vi "fgv_UI-set.vi"(7 "cmd":T1=enum."DL950 graph show", 8 "error in":errorcluster, 10 "Value":dbl, 11 "onoff":bool) -> (0 "error out":errorcluster)   [LabVIEW 2019]
uses:
  UI.ctl
  _ctrl/rw.ctl
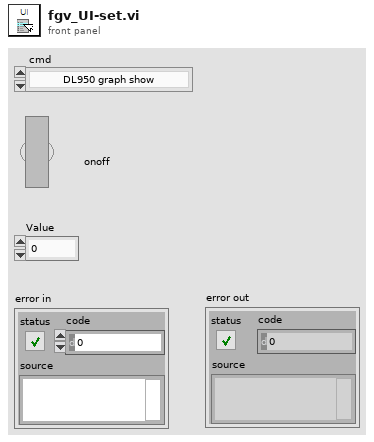
[diagram p1: front panel]
types:
  T1 = typedef "UI.ctl" = enum16{"Alarm yellow", "DL950 graph show", "DL950 graph clear", "AO value", "AO blink onoff", "Discharge relay", "Input Power", "Outpower", "Relay in1", "Relay in2", "Relay in3", "Relay in4", "Relay in5", "Relay in6", "Relay out1", "Relay out2", "Relay out3", "Relay out4", "Relay out5", "Relay out6", "Relay all off"}
  T2 = typedef "rw.ctl" = enum16{"read", "write"}
  T3 = typedef "ref_all.ctl" = cluster{"BP4610 Config":refnum<vi>, "DSP1950 Config":refnum<vi>, "2470-config":refnum<vi>, "cDAQ 9269 AO config":refnum<vi>, "cDAQ 9221 Config":refnum<vi>, "cDAQ-9467 Config":refnum<vi>, "Waveform":refnum<vi>, "DL950 wfm":refnum<vi>, "AI Graph":refnum<vi>, "AO_Wave-config":refnum<vi>, "DL950 items":refnum<vi>, "Volt":refnum<vi>, "Current":refnum<vi>, "AO_Level":refnum<vi>, "RC-Test Judgement ":refnum<vi>, "Log path":refnum<vi>, "시험명":refnum<vi>, "file renew[Hr]":refnum<vi>, "Breakdown-Spec":refnum<vi>, "paste":refnum<vi>, "copy":refnum<vi>, "DL950_config":refnum<vi>, "종료시간":refnum<vi>, "경과시간":refnum<vi>, "Apply":refnum<vi>, "DSP Config LV ":refnum<vi>, "Testconfig":refnum<vi>}
  T4 = typedef "ref.ctl" = cluster{"relay 1":refnum<vi>, "relay 2":refnum<vi>, "relay 3":refnum<vi>, "relay 4":refnum<vi>, "relay 5":refnum<vi>, "relay 6":refnum<vi>, "PoutR 1":refnum<vi>, "PoutR 2":refnum<vi>, "PoutR 3":refnum<vi>, "PoutR 4":refnum<vi>, "PoutR 5":refnum<vi>, "PoutR 6":refnum<vi>, "Discharge":refnum<vi>, "Input Pwr":refnum<vi>, "Output_HV":refnum<vi>, "AO onoff":refnum<vi>}
  T5 = typedef "ui_dev-operator.ctl" = cluster{"Operation stutus":refnum<vi>, "Test Status":refnum<vi>, "Setting":refnum<vi>, "Manual":refnum<vi>, "Main":refnum<vi>, "RCstart":refnum<vi>, "채널선택":refnum<vi>, "시험명":refnum<vi>, "Tab Control_manual":refnum<vi>, "시험 모드":refnum<vi>, "HW check":refnum<vi>, "login":refnum<vi>, "logout":refnum<vi>}
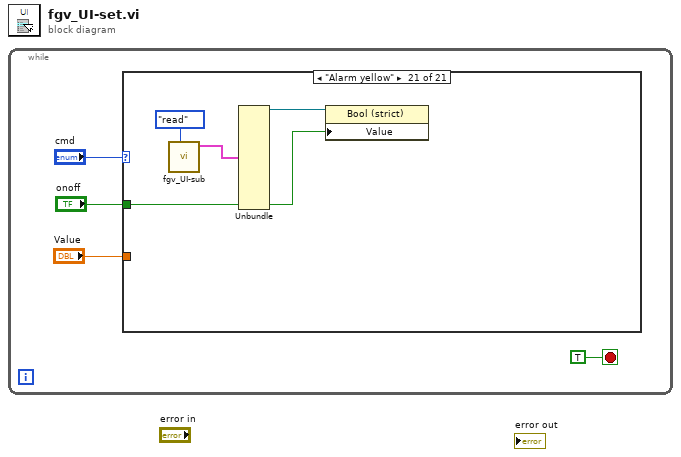
[diagram p0: block diagram]
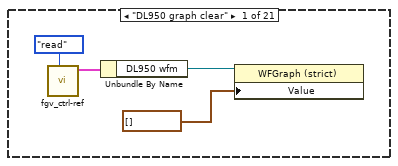
[diagram p2: hidden frame]
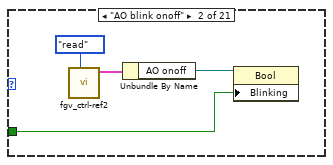
[diagram p3: hidden frame]
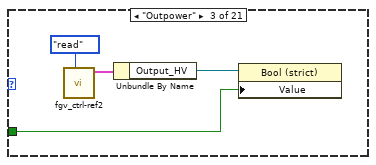
[diagram p4: hidden frame]
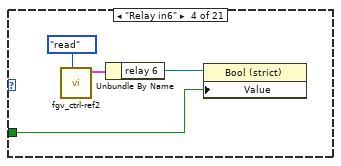
[diagram p5: hidden frame]
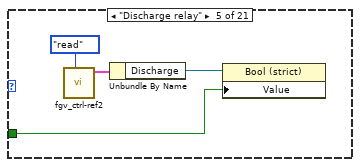
[diagram p6: hidden frame]
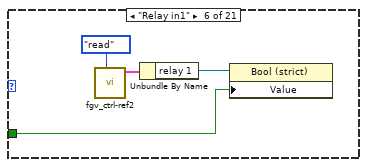
[diagram p7: hidden frame]
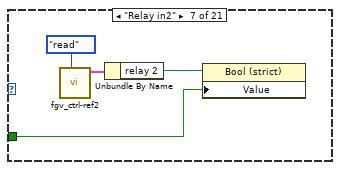
[diagram p8: hidden frame]
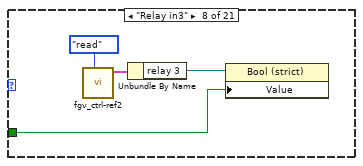
[diagram p9: hidden frame]
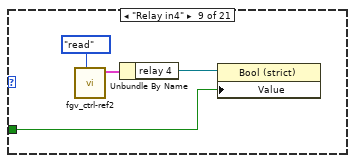
[diagram p10: hidden frame]
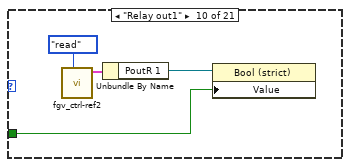
[diagram p11: hidden frame]
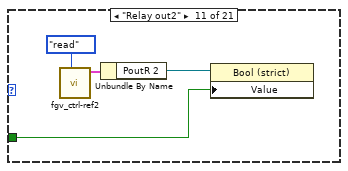
[diagram p12: hidden frame]
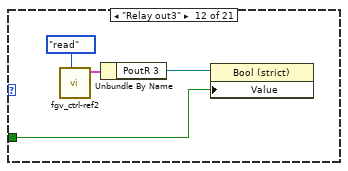
[diagram p13: hidden frame]
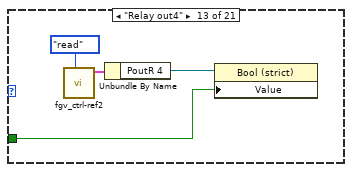
[diagram p14: hidden frame]
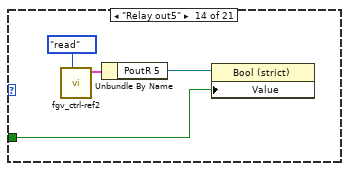
[diagram p15: hidden frame]
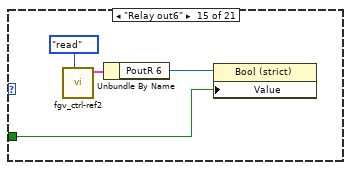
[diagram p16: hidden frame]
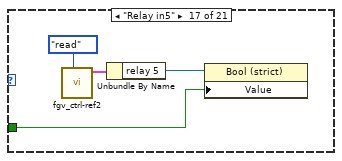
[diagram p18: hidden frame]
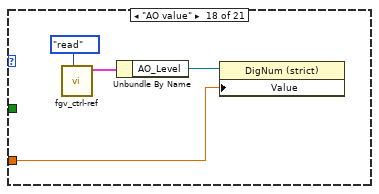
[diagram p19: hidden frame]
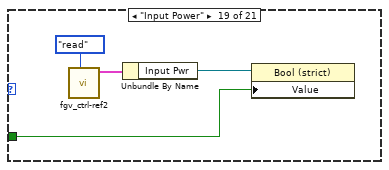
[diagram p20: hidden frame]
diagram:
  n1 = while {
    stop <- TRUE stop-if-true
    n2 = case shown="\"Alarm yellow\"" "cmd" {
      tunnel: "onoff" -> [_ w9 w13 w17 w22 w25 w29 w33 w37 w41 w45 w49 w53 w57 w61 _ w65 _ w73 _ w95]
      tunnel: "Value" -> [_ _ _ _ _ _ _ _ _ _ _ _ _ _ _ _ _ w69 _ _ _]
      frame "DL950 graph clear" {
        n3 = call "fgv_ctrl-ref.vi"("cmd"=rw."read") -> ("output cluster 2"=w7:T3)  [unwired: 9 in, 1 out]
        n4 = Unbundle By Name(w7) -> ("DL950 wfm"=w6:refnum<vi>)
        n5 = property class="WFGraph (strict)"(reference=w6, "Value"=waveform(dbl)[] []) -> ()  [unwired: 1 in, 2 out]
      }
      frame "AO blink onoff" {
        n6 = call "fgv_ctrl-ref2.vi"("cmd"=rw."read") -> ("input cluster 2"=w12:T4)  [unwired: 10 in]
        n7 = Unbundle By Name(w12) -> ("AO onoff"=w11:refnum<vi>)
        n8 = property class="Bool"(reference=w11, "Blinking"=w9) -> ()  [unwired: 1 in, 2 out]
      }
      frame "Outpower" {
        n9 = call "fgv_ctrl-ref2.vi"("cmd"=rw."read") -> ("input cluster 2"=w15:T4)  [unwired: 10 in]
        n10 = Unbundle By Name(w15) -> ("Output_HV"=w16:refnum<vi>)
        n11 = property class="Bool (strict)"(reference=w16, "Value"=w13) -> ()  [unwired: 1 in, 2 out]
      }
      frame "Relay in6" {
        n12 = call "fgv_ctrl-ref2.vi"("cmd"=rw."read") -> ("input cluster 2"=w19:T4)  [unwired: 10 in]
        n13 = Unbundle By Name(w19) -> ("relay 6"=w18:refnum<vi>)
        n14 = property class="Bool (strict)"(reference=w18, "Value"=w17) -> ()  [unwired: 1 in, 2 out]
      }
      frame "Discharge relay" {
        n15 = call "fgv_ctrl-ref2.vi"("cmd"=rw."read") -> ("input cluster 2"=w23:T4)  [unwired: 10 in]
        n16 = Unbundle By Name(w23) -> ("Discharge"=w24:refnum<vi>)
        n17 = property class="Bool (strict)"(reference=w24, "Value"=w22) -> ()  [unwired: 1 in, 2 out]
      }
      frame "Relay in1" {
        n18 = call "fgv_ctrl-ref2.vi"("cmd"=rw."read") -> ("input cluster 2"=w27:T4)  [unwired: 10 in]
        n19 = Unbundle By Name(w27) -> ("relay 1"=w26:refnum<vi>)
        n20 = property class="Bool (strict)"(reference=w26, "Value"=w25) -> ()  [unwired: 1 in, 2 out]
      }
      frame "Relay in2" {
        n21 = call "fgv_ctrl-ref2.vi"("cmd"=rw."read") -> ("input cluster 2"=w31:T4)  [unwired: 10 in]
        n22 = Unbundle By Name(w31) -> ("relay 2"=w30:refnum<vi>)
        n23 = property class="Bool (strict)"(reference=w30, "Value"=w29) -> ()  [unwired: 1 in, 2 out]
      }
      frame "Relay in3" {
        n24 = call "fgv_ctrl-ref2.vi"("cmd"=rw."read") -> ("input cluster 2"=w35:T4)  [unwired: 10 in]
        n25 = Unbundle By Name(w35) -> ("relay 3"=w34:refnum<vi>)
        n26 = property class="Bool (strict)"(reference=w34, "Value"=w33) -> ()  [unwired: 1 in, 2 out]
      }
      frame "Relay in4" {
        n27 = call "fgv_ctrl-ref2.vi"("cmd"=rw."read") -> ("input cluster 2"=w39:T4)  [unwired: 10 in]
        n28 = Unbundle By Name(w39) -> ("relay 4"=w38:refnum<vi>)
        n29 = property class="Bool (strict)"(reference=w38, "Value"=w37) -> ()  [unwired: 1 in, 2 out]
      }
      frame "Relay out1" {
        n30 = call "fgv_ctrl-ref2.vi"("cmd"=rw."read") -> ("input cluster 2"=w44:T4)  [unwired: 10 in]
        n31 = Unbundle By Name(w44) -> ("PoutR 1"=w43:refnum<vi>)
        n32 = property class="Bool (strict)"(reference=w43, "Value"=w41) -> ()  [unwired: 1 in, 2 out]
      }
      frame "Relay out2" {
        n33 = call "fgv_ctrl-ref2.vi"("cmd"=rw."read") -> ("input cluster 2"=w48:T4)  [unwired: 10 in]
        n34 = Unbundle By Name(w48) -> ("PoutR 2"=w47:refnum<vi>)
        n35 = property class="Bool (strict)"(reference=w47, "Value"=w45) -> ()  [unwired: 1 in, 2 out]
      }
      frame "Relay out3" {
        n36 = call "fgv_ctrl-ref2.vi"("cmd"=rw."read") -> ("input cluster 2"=w52:T4)  [unwired: 10 in]
        n37 = Unbundle By Name(w52) -> ("PoutR 3"=w51:refnum<vi>)
        n38 = property class="Bool (strict)"(reference=w51, "Value"=w49) -> ()  [unwired: 1 in, 2 out]
      }
      frame "Relay out4" {
        n39 = call "fgv_ctrl-ref2.vi"("cmd"=rw."read") -> ("input cluster 2"=w56:T4)  [unwired: 10 in]
        n40 = Unbundle By Name(w56) -> ("PoutR 4"=w55:refnum<vi>)
        n41 = property class="Bool (strict)"(reference=w55, "Value"=w53) -> ()  [unwired: 1 in, 2 out]
      }
      frame "Relay out5" {
        n42 = call "fgv_ctrl-ref2.vi"("cmd"=rw."read") -> ("input cluster 2"=w60:T4)  [unwired: 10 in]
        n43 = Unbundle By Name(w60) -> ("PoutR 5"=w59:refnum<vi>)
        n44 = property class="Bool (strict)"(reference=w59, "Value"=w57) -> ()  [unwired: 1 in, 2 out]
      }
      frame "Relay out6" {
        n45 = call "fgv_ctrl-ref2.vi"("cmd"=rw."read") -> ("input cluster 2"=w64:T4)  [unwired: 10 in]
        n46 = Unbundle By Name(w64) -> ("PoutR 6"=w63:refnum<vi>)
        n47 = property class="Bool (strict)"(reference=w63, "Value"=w61) -> ()  [unwired: 1 in, 2 out]
      }
      frame "DL950 graph show" {
      }
      frame "Relay in5" {
        n48 = call "fgv_ctrl-ref2.vi"("cmd"=rw."read") -> ("input cluster 2"=w67:T4)  [unwired: 10 in]
        n49 = Unbundle By Name(w67) -> ("relay 5"=w66:refnum<vi>)
        n50 = property class="Bool (strict)"(reference=w66, "Value"=w65) -> ()  [unwired: 1 in, 2 out]
      }
      frame "AO value" {
        n51 = call "fgv_ctrl-ref.vi"("cmd"=rw."read") -> ("output cluster 2"=w71:T3)  [unwired: 9 in, 1 out]
        n52 = Unbundle By Name(w71) -> ("AO_Level"=w70:refnum<vi>)
        n53 = property class="DigNum (strict)"(reference=w70, "Value"=w69) -> ()  [unwired: 1 in, 2 out]
      }
      frame "Input Power" {
        n54 = call "fgv_ctrl-ref2.vi"("cmd"=rw."read") -> ("input cluster 2"=w75:T4)  [unwired: 10 in]
        n55 = Unbundle By Name(w75) -> ("Input Pwr"=w74:refnum<vi>)
        n56 = property class="Bool (strict)"(reference=w74, "Value"=w73) -> ()  [unwired: 1 in, 2 out]
      }
      frame "Relay all off" {
        n57 = call "fgv_ctrl-ref2.vi"("cmd"=rw."read") -> ("input cluster 2"=w78:T4)  [unwired: 10 in]
        n58 = Unbundle By Name(w78) -> ("relay 1"=w79:refnum<vi>, "relay 2"=w80:refnum<vi>, "relay 3"=w81:refnum<vi>, "relay 4"=w82:refnum<vi>, "relay 5"=w83:refnum<vi>, "relay 6"=w84:refnum<vi>, "PoutR 1"=w85:refnum<vi>, "PoutR 2"=w86:refnum<vi>, "PoutR 3"=w87:refnum<vi>, "PoutR 4"=w88:refnum<vi>, "PoutR 5"=w89:refnum<vi>, "PoutR 6"=w90:refnum<vi>, "Discharge"=w91:refnum<vi>)
        n59 = Build Array(w79, w80, w81, w82, w83, w84, w85, w86, w87, w88, w89, w90, w91) -> (w92:refnum<vi>[])
        n60 = for {
          tunnel: w92 -> [w94] mode=indexing
          n61 = property class="Bool (strict)"(reference=w94, "Value"=FALSE) -> ()  [unwired: 1 in, 2 out]
        }
      }
      frame "Alarm yellow" {
        n62 = call "fgv_UI-sub.vi"("cmd"=rw."read") -> ("output cluster 2"=w97:T5)  [unwired: 9 in, 1 out]
        n63 = Unbundle(w97) -> ("Operation stutus"=w98:refnum<vi>)  [unwired: 12 out]
        n64 = property class="Bool (strict)"(reference=w98, "Value"=w95) -> ()  [unwired: 1 in, 2 out]
      }
    }
  }
